vi "Teleop.vi"(10 "Match Info":T1={"Autonomous Elapsed Seconds"=0.0, "TeleOp Elapsed Seconds"=0.0, "Disabled Elapsed Seconds"=0.0, "Visited Autonomous"=FALSE, "Visited TeleOp"=FALSE, "Visited Disabled"=FALSE, "Autonomous Settings"={"Autonomous Style"=enum."Independent", "VI Refnum"=refnum}}, 11 "Call Context":T2) -> ()   [LabVIEW 2019]
doc: "This VI is called for each TeleOp packet received from the DS where the robot is not disabled. It is often used to read from the joysticks and update I/O or to update setpoints for timed control loops. It should complete and return within 20 milliseconds or it may miss DS packets."
uses:
  <vilib>/Rock Robotics/WPI/DriverStation/WPI_DriverStationDerivedRobotMode.ctl
  <vilib>/Rock Robotics/WPI/DriverStation/WPI_DriverStationMatch Info.ctl
  <vilib>/Rock Robotics/WPI/Utilities/WPI_GetSetVariantRefNum.vi
  <vilib>/Rock Robotics/Network Tables/NT Write Boolean Array.vi
  <vilib>/Rock Robotics/Network Tables/NT Write Numeric Array.vi
  <vilib>/Rock Robotics/Network Tables/NT Read Boolean.vi
  <vilib>/Rock Robotics/Network Tables/NT Read Number.vi
  <vilib>/Rock Robotics/WPI/Solenoid/WPI_SolenoidSetEnum.vi
panel:
  out "Enabled":bool
  out "Sample Slider 0":dbl(slide) scale=0.0..5.0
  out "Sample Boolean 1":bool
  out "Sample Boolean 0":bool
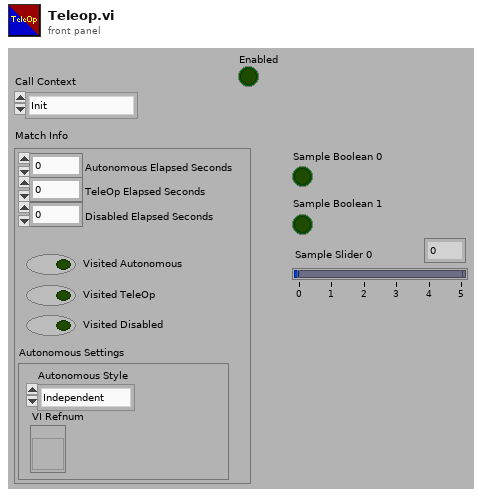
[diagram p1: front panel]
types:
  T1 = typedef "WPI_DriverStationMatch Info.ctl" = cluster{"Autonomous Elapsed Seconds":dbl, "TeleOp Elapsed Seconds":dbl, "Disabled Elapsed Seconds":dbl, "Visited Autonomous":bool, "Visited TeleOp":bool, "Visited Disabled":bool, "Autonomous Settings":cluster{"Autonomous Style":enum16{"Iterative", "Independent"}, "VI Refnum":refnum<vi>}}
  T2 = typedef "WPI_DriverStationDerivedRobotMode.ctl" = enum16{"Init", "Execute", "Stop"}
  T3 = typedef "WPI_MotorControlDeviceRef.ctl" = cluster{"DeviceStatus":errorcluster, "Type":T4, "PWM":cluster{"PWM Channel":T5, "DeadBand":T6}, "CAN":cluster{"Device Number":u8, "SetOutput VI Ref":variant, "GetOutput VI Ref":variant, "Enable VI Ref":variant, "Disable VI Ref":variant, "Data":variant}, "Invert":bool, "DIO PWM":cluster{"PWM \"Enable\" Channel":T5, "DIOChannel":T7, "PWM Rate":dbl}}
  T4 = typedef "WPI_MotorControlType.ctl" = enum16{"PWM", "CAN", "DIO PWM"}
  T5 = typedef "FPGA_DIOPWMChannel.ctl" = enum8{"PWM 0", "PWM 1", "PWM 2", "PWM 3", "PWM 4", "PWM 5", "PWM 6", "PWM 7", "PWM 8", "PWM 9", "PWM MXP 0", "PWM MXP 1", "PWM MXP 2", "PWM MXP 3", "PWM MXP 4", "PWM MXP 5", "PWM MXP 6", "PWM MXP 7", "PWM MXP 8", "PWM MXP 9", "Invalid"}
  T6 = typedef "WPI_PWMDeadband.ctl" = cluster{"Name":string, "maxPositivePwm":i32, "minPositivePwm":i32, "centerPwm":i32, "maxNegativePwm":i32, "minNegativePwm":i32, "angularRange":u16}
  T7 = typedef "FPGA_DIOChannel.ctl" = enum8{"DIO 0", "DIO 1", "DIO 2", "DIO 3", "DIO 4", "DIO 5", "DIO 6", "DIO 7", "DIO 8", "DIO 9", "DIO MXP 0", "DIO MXP 1", "DIO MXP 2", "DIO MXP 3", "DIO MXP 4", "DIO MXP 5", "DIO MXP 6", "DIO MXP 7", "DIO MXP 8", "DIO MXP 9", "DIO MXP 10", "DIO MXP 11", "DIO MXP 12", "DIO MXP 13", "DIO MXP 14", "DIO MXP 15", "SPI Port CS1", "SPI Port CS2", "SPI Port CS3", "SPI Port MISO", "SPI Port MOSI", "Invalid"}
  T8 = typedef "WPI_JoystickDevRef.ctl" = cluster{"Device":T9}
  T9 = typedef "WPI_JoystickDeviceEnum.ctl" = enum16{"USB 0", "USB 1", "USB 2", "USB 3", "USB 4", "USB 5"}
  T10 = typedef "WPI_RobotDriveDevRef.ctl" = cluster{"DevStatus":errorcluster, "Motors[]":T3[], "Square Inputs":bool, "Max Output":dbl}
  T11 = typedef "WPI_SolenoidDevRef.ctl" = cluster{"DevStatus":errorcluster, "Pneumatics Control Module":u8, "Forward Solenoid Channel":T12, "Reverse Solenoid Channel":T12}
  T12 = typedef "WPI_SolenoidChannel.ctl" = enum8{"Solenoid 0", "Solenoid 1", "Solenoid 2", "Solenoid 3", "Solenoid 4", "Solenoid 5", "Solenoid 6", "Solenoid 7", "Invalid"}
  T13 = typedef "WPI_CompressorDevRef.ctl" = cluster{"DevStatus":errorcluster, "Pneumatics Control Module":u8}
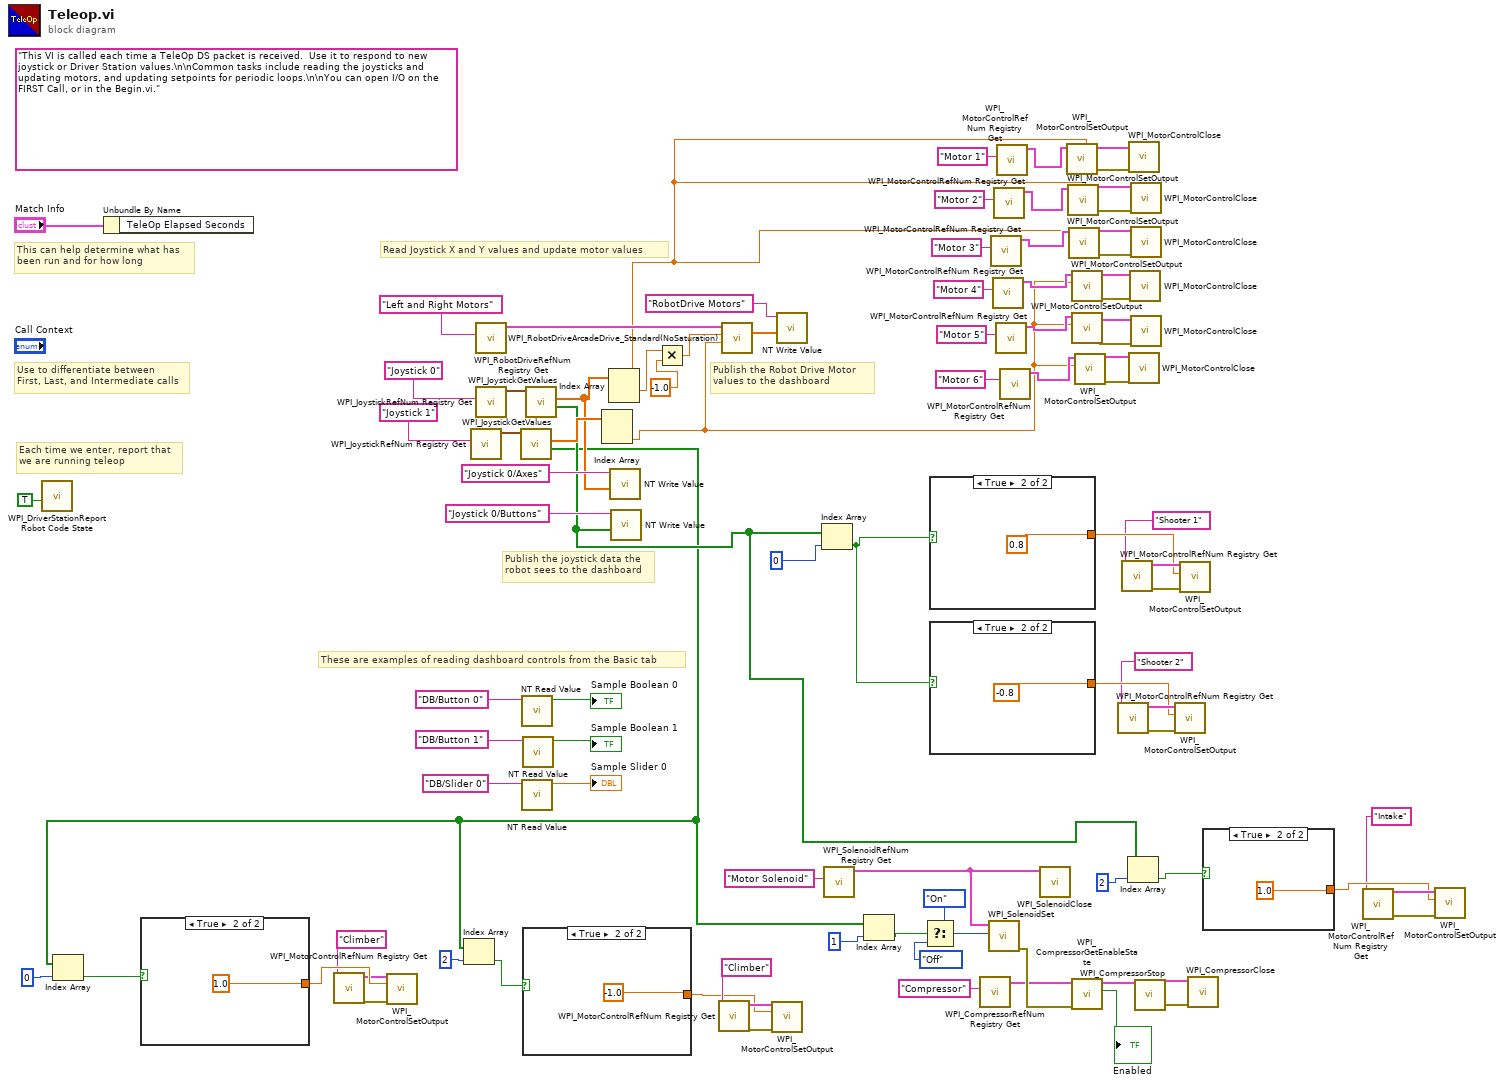
[diagram p0: block diagram]
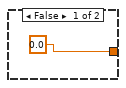
[diagram p2: hidden frame]
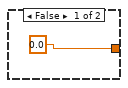
[diagram p3: hidden frame]
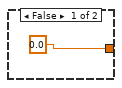
[diagram p4: hidden frame]
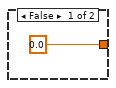
[diagram p5: hidden frame]
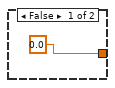
[diagram p6: hidden frame]
diagram:
  (unwired) "This VI is called each time a TeleOp DS packet is received.  Use it to respond to new joystick or Driver Station values.\n\nCommon tasks include reading the joysticks and updating motors, and updating setpoints for periodic loops.\n\nYou can open I/O on the FIRST Call, or in the Begin.vi."
  # "These are examples of reading dashboard controls from the Basic tab"
  # "Publish the Robot Drive Motor\nvalues to the dashboard"
  # "Publish the joystick data the\nrobot sees to the dashboard"
  # "Each time we enter, report that\nwe are running teleop"
  # "Use to differentiate between\nFirst, Last, and Intermediate calls"
  # "This can help determine what has\nbeen run and for how long"
  # "Read Joystick X and Y values and update motor values"
  n1 = call <vilib>:"WPI_DriverStationReport Robot Code State.vi"("TeleOp"=TRUE ("Autonomous")) -> ()  [unwired: 10 in, 1 out]
  n2 = Unbundle By Name("Match Info") -> ()  [unwired: 1 out]
  n3 = call <vilib>:"WPI_MotorControlRefNum Registry Get.vi"("refnum name"="Climber") -> ("error out"=w18:errorcluster, "MotorControlDevRef"=w19:T3)  [unwired: 9 in]
  n4 = call <vilib>:"WPI_JoystickRefNum Registry Get.vi"("refnum name"="Joystick 1") -> ("JoystickDevRef"=w75:T8)  [unwired: 1 in, 9 out]
  n5 = call <vilib>:"WPI_RobotDriveRefNum Registry Get.vi"("refnum name"="Left and Right Motors") -> ("RobotDriveDevRef"=w90:T10)  [unwired: 1 in, 9 out]
  n6 = call <vilib>:"WPI_JoystickRefNum Registry Get.vi"("refnum name"="Joystick 0") -> ("JoystickDevRef"=w88:T8)  [unwired: 1 in, 9 out]
  n7 = call <vilib>:"WPI_JoystickGetValues.vi"("JoystickDevRef"=w75) -> ("Buttons"=w5:bool[], "Axes"=w74:dbl[])  [unwired: 6 in, 3 out]
  n8 = Index Array(array=w5, index=0) -> (element=w9:bool)
  n9 = case shown="True" w9 {
    tunnel: [0.0 1.0] -> w20
    frame False {
    }
    frame True {
    }
  }
  n10 = call <vilib>:"WPI_MotorControlSetOutput.vi"("error in (no error)"=w18, "Output"=w20, "MotorControlDevRef"=w19) -> ()  [unwired: 6 in, 3 out]
  n11 = Index Array(array=w5, index=2) -> (element=w12:bool)
  n12 = call-poly <vilib>:"NT Read Value.vi"("Name"="DB/Button 0" ("refnum name")) -> ("Boolean"=→"Sample Boolean 0":bool)  [unwired: 9 in, 1 out]
  n13 = call-poly <vilib>:"NT Read Value.vi"("Name"="DB/Slider 0" ("refnum name")) -> ("Numeric"=→"Sample Slider 0":dbl)  [unwired: 9 in, 1 out]
  n14 = call-poly <vilib>:"NT Read Value.vi"("Name"="DB/Button 1" ("refnum name")) -> ("Boolean"=→"Sample Boolean 1":bool)  [unwired: 9 in, 1 out]
  n15 = case shown="True" w12 {
    tunnel: [0.0 -1.0] -> w13
    frame False {
    }
    frame True {
    }
  }
  n16 = call <vilib>:"WPI_JoystickGetValues.vi"("JoystickDevRef"=w88) -> ("Buttons"=w10:bool[], "Axes"=w73:dbl[])  [unwired: 6 in, 3 out]
  n17 = Index Array(array=w74) -> (element #2=w4:dbl)  [unwired: 2 in, 1 out]
  n18 = Index Array(array=w73) -> (element #1=w3:dbl)  [unwired: 2 in, 1 out]
  n19 = call-poly <vilib>:"NT Write Value.vi"("Numeric Array"=w73, "Name"="Joystick 0/Axes") -> ()  [unwired: 9 in, 1 out]
  n20 = call-poly <vilib>:"NT Write Value.vi"("Boolean Array"=w10, "Name"="Joystick 0/Buttons") -> ()  [unwired: 9 in, 1 out]
  n21 = Multiply(x=w3, y=-1.0) -> (x*y=w2:dbl)
  n22 = call <vilib>:"WPI_MotorControlRefNum Registry Get.vi"("refnum name"="Climber") -> ("error out"=w15:errorcluster, "MotorControlDevRef"=w16:T3)  [unwired: 9 in]
  n23 = call <vilib>:"WPI_RobotDriveArcadeDrive_Standard(NoSaturation).vi"("Y axis value"=w4, "X axis value"=w2, "RobotDriveDevRef"=w90) -> ("Motor Values"=w78:dbl[])  [unwired: 1 in, 7 out]
  n24 = call <vilib>:"WPI_MotorControlSetOutput.vi"("error in (no error)"=w15, "Output"=w13, "MotorControlDevRef"=w16) -> ()  [unwired: 6 in, 3 out]
  n25 = call-poly <vilib>:"NT Write Value.vi"("Numeric Array"=w78, "Name"="RobotDrive Motors") -> ()  [unwired: 9 in, 1 out]
  n26 = Index Array(array=w10, index=0) -> (element=w71:bool)
  n27 = call <vilib>:"WPI_SolenoidRefNum Registry Get.vi"("refnum name"="Motor Solenoid") -> ("SolenoidDevRef"=w35:T11)  [unwired: 9 in, 1 out]
  n28 = Index Array(array=w5, index=1) -> (element=w7:bool)
  n29 = Select(t=enum16{"On"}."On", s=w7, f=enum16{"Off"}."Off") -> (s? t:f=w38:u16)
  n30 = case shown="True" w71 {
    tunnel: [0.0 0.8] -> w66
    frame False {
    }
    frame True {
    }
  }
  n31 = case shown="True" w71 {
    tunnel: [0.0 -0.8] -> w65
    frame False {
    }
    frame True {
    }
  }
  n32 = call <vilib>:"WPI_CompressorRefNum Registry Get.vi"("refnum name"="Compressor") -> ("CompressorDevRef"=w30:T13)  [unwired: 9 in, 1 out]
  n33 = call-poly <vilib>:"WPI_SolenoidSet.vi"("Value"=w38, "SolenoidDevRef"=w35) -> ("error out"=w37:errorcluster)  [unwired: 8 in, 1 out]
  n34 = call <vilib>:"WPI_MotorControlRefNum Registry Get.vi"("refnum name"="Motor 3") -> ("MotorControlDevRef"=w53:T3)  [unwired: 9 in, 1 out]
  n35 = call <vilib>:"WPI_MotorControlRefNum Registry Get.vi"("refnum name"="Motor 4") -> ("MotorControlDevRef"=w54:T3)  [unwired: 9 in, 1 out]
  n36 = call <vilib>:"WPI_MotorControlRefNum Registry Get.vi"("refnum name"="Motor 2") -> ("MotorControlDevRef"=w52:T3)  [unwired: 9 in, 1 out]
  n37 = call <vilib>:"WPI_MotorControlRefNum Registry Get.vi"("refnum name"="Motor 5") -> ("MotorControlDevRef"=w55:T3)  [unwired: 9 in, 1 out]
  n38 = call <vilib>:"WPI_MotorControlRefNum Registry Get.vi"("refnum name"="Motor 1") -> ("MotorControlDevRef"=w51:T3)  [unwired: 9 in, 1 out]
  n39 = call <vilib>:"WPI_MotorControlRefNum Registry Get.vi"("refnum name"="Motor 6") -> ("MotorControlDevRef"=w56:T3)  [unwired: 9 in, 1 out]
  n40 = call <vilib>:"WPI_SolenoidClose.vi"("SolenoidDevRef"=w35) -> ()  [unwired: 10 in, 1 out]
  n41 = call <vilib>:"WPI_MotorControlSetOutput.vi"("Output"=w3, "MotorControlDevRef"=w51) -> ("error out"=w39:errorcluster, "MotorControlDevRef"=w50:T3)  [unwired: 7 in, 1 out]
  n42 = call <vilib>:"WPI_MotorControlSetOutput.vi"("Output"=w3, "MotorControlDevRef"=w52) -> ("error out"=w41:errorcluster, "MotorControlDevRef"=w40:T3)  [unwired: 7 in, 1 out]
  n43 = call <vilib>:"WPI_MotorControlSetOutput.vi"("Output"=w3, "MotorControlDevRef"=w53) -> ("error out"=w42:errorcluster, "MotorControlDevRef"=w43:T3)  [unwired: 7 in, 1 out]
  n44 = call <vilib>:"WPI_MotorControlSetOutput.vi"("Output"=w4, "MotorControlDevRef"=w54) -> ("error out"=w44:errorcluster, "MotorControlDevRef"=w45:T3)  [unwired: 7 in, 1 out]
  n45 = call <vilib>:"WPI_MotorControlSetOutput.vi"("Output"=w4, "MotorControlDevRef"=w55) -> ("error out"=w47:errorcluster, "MotorControlDevRef"=w46:T3)  [unwired: 7 in, 1 out]
  n46 = call <vilib>:"WPI_CompressorGetEnableState.vi"("error in (no error)"=w37, "CompressorDevRef"=w30) -> ("Enabled"=→"Enabled":bool, "CompressorDevRef"=w33:T13)  [unwired: 6 in, 2 out]
  n47 = call <vilib>:"WPI_MotorControlSetOutput.vi"("Output"=w4, "MotorControlDevRef"=w56) -> ("error out"=w48:errorcluster, "MotorControlDevRef"=w49:T3)  [unwired: 7 in, 1 out]
  n48 = call <vilib>:"WPI_MotorControlRefNum Registry Get.vi"("refnum name"="Shooter 2") -> ("error out"=w68:errorcluster, "MotorControlDevRef"=w70:T3)  [unwired: 9 in]
  n49 = call <vilib>:"WPI_MotorControlRefNum Registry Get.vi"("refnum name"="Shooter 1") -> ("error out"=w67:errorcluster, "MotorControlDevRef"=w69:T3)  [unwired: 9 in]
  n50 = Index Array(array=w10, index=2) -> (element=w26:bool)
  n51 = call <vilib>:"WPI_MotorControlClose.vi"("error in"=w39, "MotorControlDevRef"=w50) -> ()  [unwired: 9 in, 1 out]
  n52 = call <vilib>:"WPI_MotorControlClose.vi"("error in"=w48, "MotorControlDevRef"=w49) -> ()  [unwired: 9 in, 1 out]
  n53 = call <vilib>:"WPI_MotorControlClose.vi"("error in"=w44, "MotorControlDevRef"=w45) -> ()  [unwired: 9 in, 1 out]
  n54 = call <vilib>:"WPI_MotorControlClose.vi"("error in"=w41, "MotorControlDevRef"=w40) -> ()  [unwired: 9 in, 1 out]
  n55 = call <vilib>:"WPI_MotorControlClose.vi"("error in"=w42, "MotorControlDevRef"=w43) -> ()  [unwired: 9 in, 1 out]
  n56 = call <vilib>:"WPI_MotorControlClose.vi"("error in"=w47, "MotorControlDevRef"=w46) -> ()  [unwired: 9 in, 1 out]
  n57 = call <vilib>:"WPI_CompressorStop.vi"("CompressorDevRef"=w33) -> ("error out"=w31:errorcluster, "CompressorDevRef"=w32:T13)  [unwired: 9 in]
  n58 = call <vilib>:"WPI_MotorControlSetOutput.vi"("error in (no error)"=w68, "Output"=w65, "MotorControlDevRef"=w70) -> ()  [unwired: 6 in, 3 out]
  n59 = call <vilib>:"WPI_MotorControlSetOutput.vi"("error in (no error)"=w67, "Output"=w66, "MotorControlDevRef"=w69) -> ()  [unwired: 6 in, 3 out]
  n60 = call <vilib>:"WPI_CompressorClose.vi"("error in (no error)"=w31, "CompressorDevRef"=w32) -> ()  [unwired: 9 in, 1 out]
  n61 = case shown="True" w26 {
    tunnel: [0.0 1.0] -> w22
    frame False {
    }
    frame True {
    }
  }
  n62 = call <vilib>:"WPI_MotorControlRefNum Registry Get.vi"("refnum name"="Intake") -> ("error out"=w23:errorcluster, "MotorControlDevRef"=w24:T3)  [unwired: 9 in]
  n63 = call <vilib>:"WPI_MotorControlSetOutput.vi"("error in (no error)"=w23, "Output"=w22, "MotorControlDevRef"=w24) -> ()  [unwired: 6 in, 3 out]
